vi "Write Angle.vi"(8 "error in (no error)":errorcluster, 10 "Angle":dbl, 11 "Water Tunnel Results in":refnum<class "Water Tunnel Results.lvclass">) -> (0 "error out":errorcluster, 3 "Water Tunnel Results out":refnum<class "Water Tunnel Results.lvclass">)   [LabVIEW 2019, in "Results.lvlib" / "Water Tunnel Results.lvclass"]
uses:
  Water Tunnel Results.lvclass
  Water Tunnel Results.lvclass/Water Tunnel Results.ctl
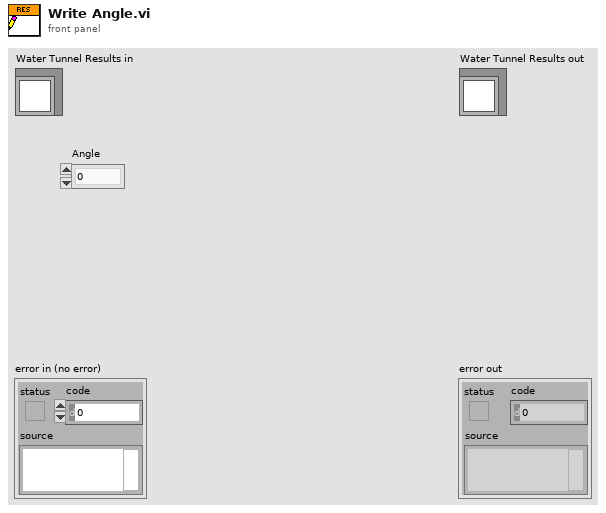
[diagram p1: front panel]
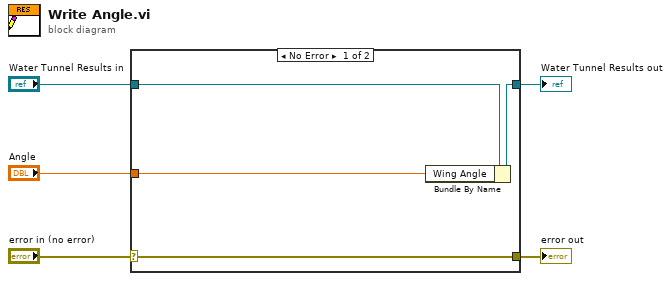
[diagram p0: block diagram]
diagram:
  n1 = case shown="No Error" "error in (no error)" {
    selector: "error in (no error)" -> [w9 w10]
    tunnel: [w9 w10] -> w4
    tunnel: [w7 w11] -> w2
    tunnel: "Water Tunnel Results in" -> [w8 w11]
    tunnel: "Angle" -> [w6 _]
    frame No Error {
      n2 = Bundle By Name(cluster=w8, "Wing Angle"=w6) -> (w7:refnum<class "Water Tunnel Results.lvclass">)
    }
    frame Error {
    }
  }
  "error out" <- w4
  "Water Tunnel Results out" <- w2
